vi "ultrasonic_global.vi"() -> ()   [LabVIEW 2017]
panel:
  in  "Right Object Range":dbl
  in  "Left Object Range":dbl
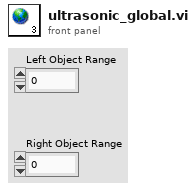
[diagram p1: front panel]
diagram:
